vi "Calculate Cubic Bezier.vi"(7 "Iterations":i32=10000, 9 "error in (no error)":errorcluster, 11 "Points":T1[](array[typedef])) -> (1 "error out":errorcluster, 2 "Y":dbl[](array[numeric]), 3 "X":dbl[](array[numeric]))   [LabVIEW 2019, in "Tool Path.lvclass"]
uses:
  Tool Path.lvclass
  Parse/PathCommands/Point.ctl
  Parse/PathCommands/PathCommands.lvclass
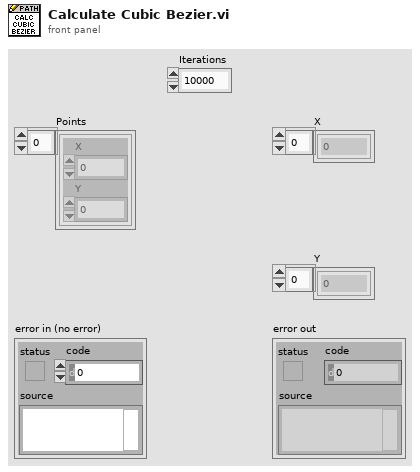
[diagram p1: front panel]
types:
  T1 = typedef "PathCommands.lvclass/Point.ctl" = cluster{"X":dbl, "Y":dbl}
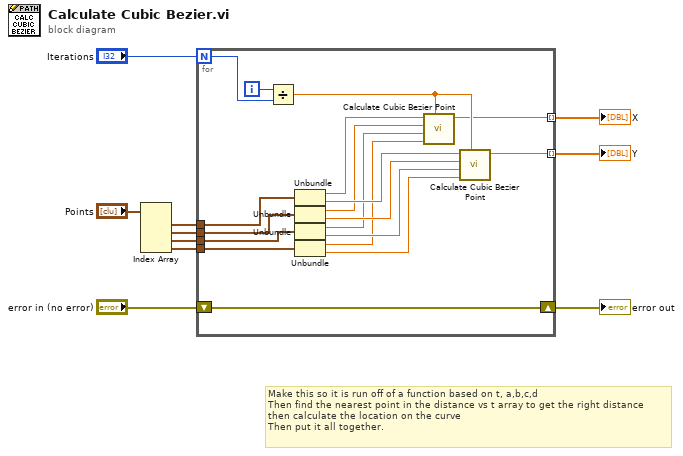
[diagram p0: block diagram]
diagram:
  # "Make this so it is run off of a function based on t, a,b,c,d\nThen find the nearest point in the distance vs t array to get the right distance\nthen calculate the location on the curve\nThen put it all together."
  n1 = Index Array(array="Points") -> (element #1=w7:T1, element #2=w6:T1, element #3=w5:T1, element #4=w4:T1)  [unwired: 4 in]
  n2 = for {
    N: "Iterations" -> [w26]
    shift-right: [w28] -> w9
    shift-left: "error in (no error)" -> [w28]
    tunnel: w7 -> [w13]
    tunnel: w6 -> [w12]
    tunnel: w5 -> [w11]
    tunnel: w4 -> [w24]
    tunnel: [w23] -> w2 mode=indexing
    tunnel: [w22] -> w1 mode=indexing
    i -> [w27]
    n3 = Divide(x=w27, y=w26) -> (x/y=w25:dbl)
    n4 = Unbundle(w13) -> ("X"=w14:dbl, "Y"=w18:dbl)
    n5 = Unbundle(w12) -> ("X"=w17:dbl, "Y"=w19:dbl)
    n6 = Unbundle(w11) -> ("X"=w16:dbl, "Y"=w20:dbl)
    n7 = Unbundle(w24) -> ("X"=w15:dbl, "Y"=w21:dbl)
    n8 = call "Calculate Cubic Bezier Point.vi"("t"=w25, "d"=w15, "c"=w16, "b"=w17, "a"=w14) -> ("f(t)"=w23:dbl)  [unwired: 6 in]
    n9 = call "Calculate Cubic Bezier Point.vi"("t"=w25, "d"=w21, "c"=w20, "b"=w19, "a"=w18) -> ("f(t)"=w22:dbl)  [unwired: 6 in]
  }
  "error out" <- w9
  "X" <- w2
  "Y" <- w1
